vi "发送数组-ccp转换序列.vi"(8 "标定站地址":u32=1 format="%x", 9 "初始地址":u32=15360 format="%x", 10 "输入数组":T2(array[cluster]), 11 "是否剩余":bool) -> (2 "输出数组":T1(array[cluster]) {"Data7" format="%x"; "Data6" format="%x"; "Data5" format="%x"; "Data4" format="%x"; "Data3" format="%x"; "Data2" format="%x"; "Data1" format="%x"; "Data0" format="%x"})   [LabVIEW 2016]
panel:
  in  "CCP命令":u16(ring) items=["CONNECT"=1, "SET_MTA"=2, "DNLOAD"=3, "UPLOAD"=4, "DISCONNECT"=7, "START_STOP_ALL"=8, "SHORT_UPLOAD"=15, "GET_DAQ_SIZE"=20, "SET_DAQ_PTR"=21, "WRITE_DAQ"=22, "EXCHANGE_ID"=23, "DNLOAD6"=35, "UNLOACK"=19, "SET_S_STATUS"=12, "GET_S_STATUS"=13, "SET_CAL_PAGE"=17, "GET_CAL_PAGE"=9, "GET_SEED"=18]
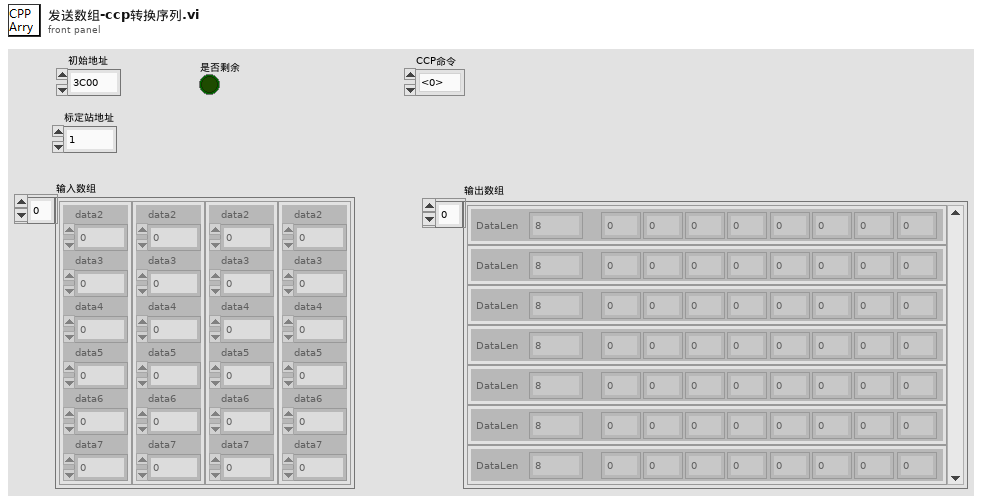
[diagram p1: front panel]
types:
  T1 = cluster{"Data0":u8, "Data1":u8, "Data2":u8, "Data3":u8, "Data4":u8, "Data5":u8, "Data6":u8, "Data7":u8, "DataLen":u8}[]
  T2 = cluster{"data2":u8, "data3":u8, "data4":u8, "data5":u8, "data6":u8, "data7":u8}[]
  T3 = cluster{"Data0":u8, "Data1":u8, "Data2":u8, "Data3":u8, "Data4":u8, "Data5":u8, "Data6":u8, "Data7":u8, "DataLen":u8}
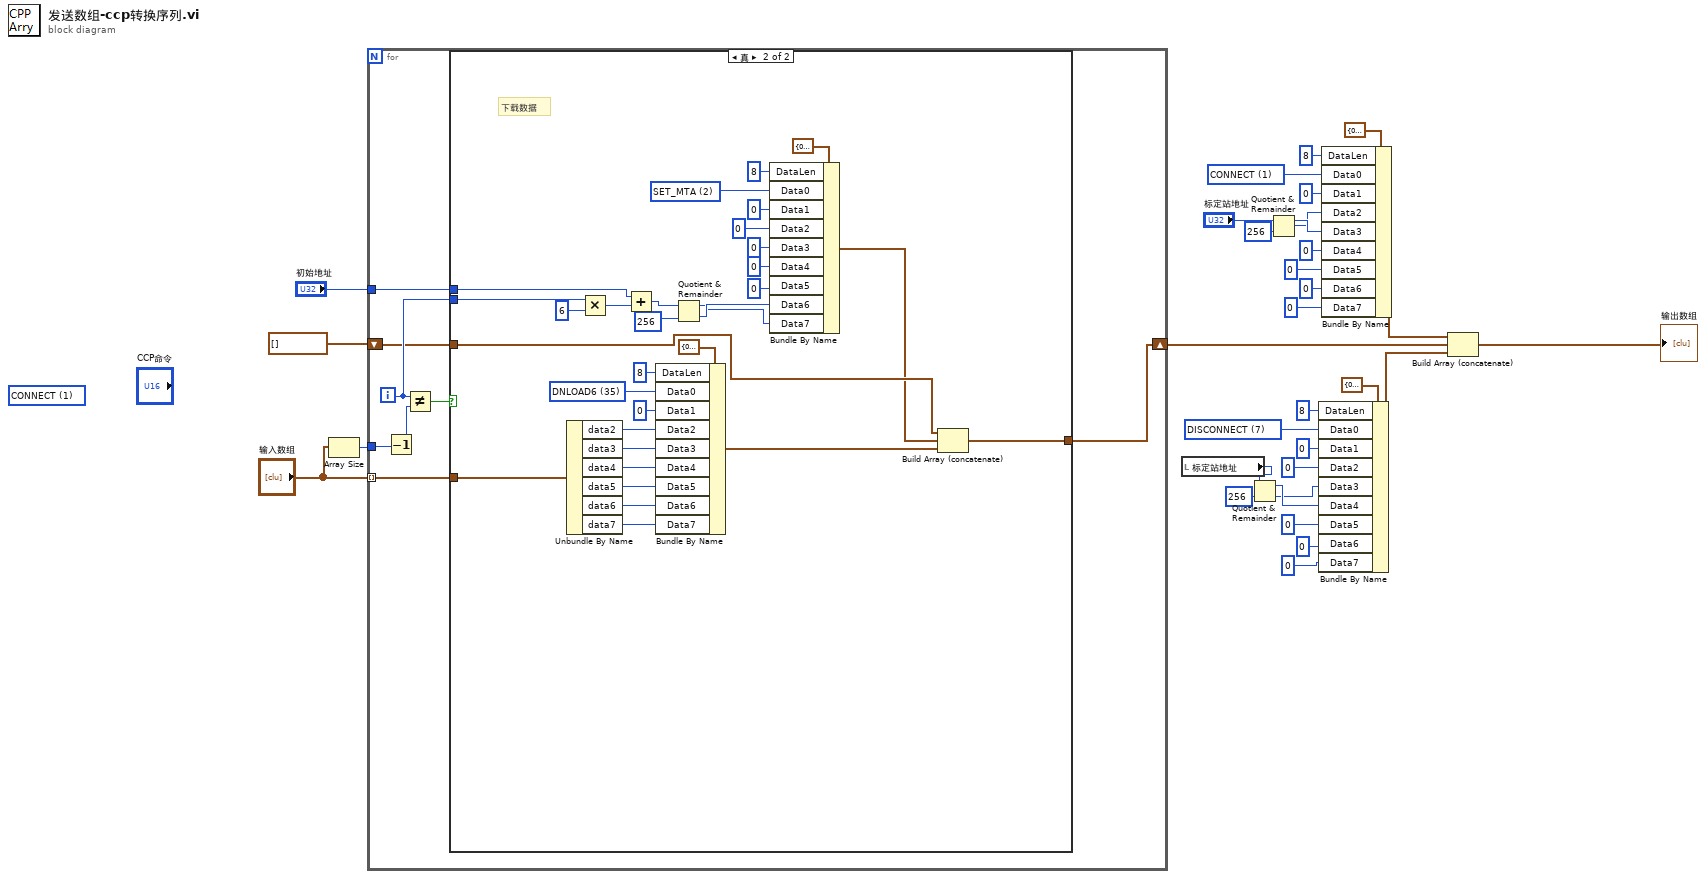
[diagram p0: block diagram]
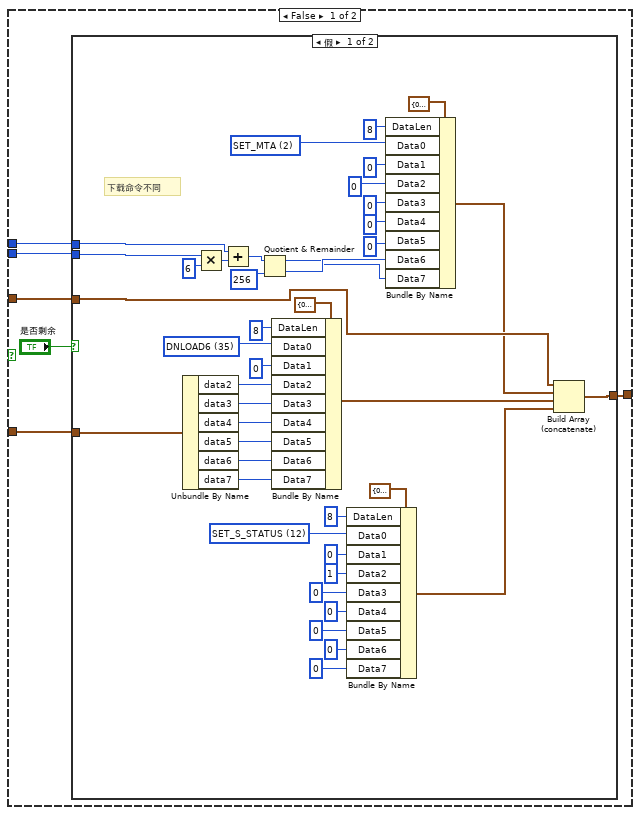
[diagram p2: hidden frame]
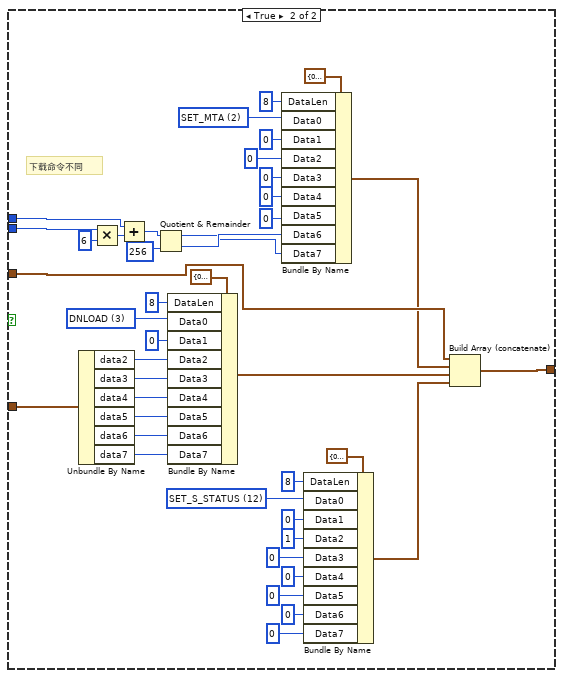
[diagram p3: hidden frame]
diagram:
  w14 = u8 7 items=["CONNECT"=1, "SET_MTA"=2, "DNLOAD"=3, "UPLOAD"=4, "DISCONNECT"=7, "START_STOP_ALL"=8, "SHORT_UPLOAD"=15, "GET_DAQ_SIZE"=20, "SET_DAQ_PTR"=21, "WRITE_DAQ"=22, "EXCHANGE_ID"=23, "DNLOAD6"=35, "UNLOACK"=19, "SET_S_STATUS"=12, "GET_S_STATUS"=13, "SET_CAL_PAGE"=17, "GET_CAL_PAGE"=9, "GET_SEED"=18] ("下拉列表")
  w26 = u8 1 items=["CONNECT"=1, "SET_MTA"=2, "DNLOAD"=3, "UPLOAD"=4, "DISCONNECT"=7, "START_STOP_ALL"=8, "SHORT_UPLOAD"=15, "GET_DAQ_SIZE"=20, "SET_DAQ_PTR"=21, "WRITE_DAQ"=22, "EXCHANGE_ID"=23, "DNLOAD6"=35, "UNLOACK"=19, "SET_S_STATUS"=12, "GET_S_STATUS"=13, "SET_CAL_PAGE"=17, "GET_CAL_PAGE"=9, "GET_SEED"=18] ("下拉列表")
  (unwired) u8 1 items=["CONNECT"=1, "SET_MTA"=2, "DNLOAD"=3, "UPLOAD"=4, "DISCONNECT"=7, "START_STOP_ALL"=8, "SHORT_UPLOAD"=15, "GET_DAQ_SIZE"=20, "SET_DAQ_PTR"=21, "WRITE_DAQ"=22, "EXCHANGE_ID"=23, "DNLOAD6"=35, "UNLOACK"=19, "SET_S_STATUS"=12, "GET_S_STATUS"=13, "SET_CAL_PAGE"=17, "GET_CAL_PAGE"=9, "GET_SEED"=18] ("下拉列表")
  n1 = Array Size(array="输入数组") -> (size(s)=w31:i32)
  n2 = for {
    tunnel: "输入数组" -> [w40] mode=indexing
    tunnel: w31 -> [w34]
    tunnel: "初始地址" -> [w37]
    shift-right: [w35] -> w8
    shift-left: T1 [] -> [w36]
    i -> [w38]
    n3 = Decrement(x=w34) -> (x-1=w33:i32)
    n4 = Not Equal?(x=w38, y=w33) -> (x != y?=w39:bool)
    n5 = case shown="真" w39 {
      tunnel: w40 -> [w45 w161]
      tunnel: w38 -> [w43 w160]
      tunnel: w37 -> [w42 w159]
      tunnel: w36 -> [w44 w158]
      tunnel: [w46 w157] -> w35
      frame False {
        n6 = case shown="假" "是否剩余" {
          tunnel: w45 -> [w87 w130]
          tunnel: w43 -> [w85 w129]
          tunnel: w42 -> [w84 w128]
          tunnel: w44 -> [w86 w127]
          tunnel: [w88 w126] -> w46
          frame False {
            w55 = u8 12 items=["CONNECT"=1, "SET_MTA"=2, "DNLOAD"=3, "UPLOAD"=4, "DISCONNECT"=7, "START_STOP_ALL"=8, "SHORT_UPLOAD"=15, "GET_DAQ_SIZE"=20, "SET_DAQ_PTR"=21, "WRITE_DAQ"=22, "EXCHANGE_ID"=23, "DNLOAD6"=35, "UNLOACK"=19, "SET_S_STATUS"=12, "GET_S_STATUS"=13, "SET_CAL_PAGE"=17, "GET_CAL_PAGE"=9, "GET_SEED"=18] ("下拉列表")
            w59 = u8 35 items=["CONNECT"=1, "SET_MTA"=2, "DNLOAD"=3, "UPLOAD"=4, "DISCONNECT"=7, "START_STOP_ALL"=8, "SHORT_UPLOAD"=15, "GET_DAQ_SIZE"=20, "SET_DAQ_PTR"=21, "WRITE_DAQ"=22, "EXCHANGE_ID"=23, "DNLOAD6"=35, "UNLOACK"=19, "SET_S_STATUS"=12, "GET_S_STATUS"=13, "SET_CAL_PAGE"=17, "GET_CAL_PAGE"=9, "GET_SEED"=18] ("下拉列表")
            w58 = u8 2 items=["CONNECT"=1, "SET_MTA"=2, "DNLOAD"=3, "UPLOAD"=4, "DISCONNECT"=7, "START_STOP_ALL"=8, "SHORT_UPLOAD"=15, "GET_DAQ_SIZE"=20, "SET_DAQ_PTR"=21, "WRITE_DAQ"=22, "EXCHANGE_ID"=23, "DNLOAD6"=35, "UNLOACK"=19, "SET_S_STATUS"=12, "GET_S_STATUS"=13, "SET_CAL_PAGE"=17, "GET_CAL_PAGE"=9, "GET_SEED"=18] ("下拉列表")
            # "下载命令不同"
            n7 = Unbundle By Name(w87) -> ("data2"=w82:u8, "data3"=w81:u8, "data4"=w80:u8, "data5"=w79:u8, "data6"=w78:u8, "data7"=w77:u8)
            n8 = Multiply(x=w85, y=6) -> (x*y=w72:i32)
            n9 = Add(x=w84, y=w72) -> (x+y=w71:u32)
            n10 = Quotient & Remainder(x=w71, y=u32 256) -> (x-y*floor(x/y)=w63:u32, floor(x/y)=w64:u32)
            n11 = Bundle By Name(cluster=T3 {"Data0"=0, "Data1"=0, "Data2"=0, "Data3"=0, "Data4"=0, "Data5"=0, "Data6"=0, "Data7"=0, "DataLen"=8} ("簇 2"), "DataLen"=u8 8, "Data0"=w59, "Data1"=u8 0, "Data2"=w82, "Data3"=w81, "Data4"=w80, "Data5"=w79, "Data6"=w78, "Data7"=w77) -> (w74:T3)
            n12 = Bundle By Name(cluster=T3 {"Data0"=0, "Data1"=0, "Data2"=0, "Data3"=0, "Data4"=0, "Data5"=0, "Data6"=0, "Data7"=0, "DataLen"=8} ("簇 2"), "DataLen"=u8 8, "Data0"=w55, "Data1"=u8 0, "Data2"=u8 1, "Data3"=u8 0, "Data4"=u8 0, "Data5"=u8 0, "Data6"=u8 0, "Data7"=u8 0) -> (w47:T3)
            n13 = Bundle By Name(cluster=T3 {"Data0"=0, "Data1"=0, "Data2"=0, "Data3"=0, "Data4"=0, "Data5"=0, "Data6"=0, "Data7"=0, "DataLen"=8} ("簇 2"), "DataLen"=u8 8, "Data0"=w58, "Data1"=u8 0, "Data2"=u8 0, "Data3"=u8 0, "Data4"=u8 0, "Data5"=u8 0, "Data6"=w64, "Data7"=w63) -> (w60:T3)
            n14 = Build Array (concatenate)(w86, w60, w74, w47) -> (w88:T1)
          }
          frame True {
            w97 = u8 12 items=["CONNECT"=1, "SET_MTA"=2, "DNLOAD"=3, "UPLOAD"=4, "DISCONNECT"=7, "START_STOP_ALL"=8, "SHORT_UPLOAD"=15, "GET_DAQ_SIZE"=20, "SET_DAQ_PTR"=21, "WRITE_DAQ"=22, "EXCHANGE_ID"=23, "DNLOAD6"=35, "UNLOACK"=19, "SET_S_STATUS"=12, "GET_S_STATUS"=13, "SET_CAL_PAGE"=17, "GET_CAL_PAGE"=9, "GET_SEED"=18] ("下拉列表")
            w101 = u8 3 items=["CONNECT"=1, "SET_MTA"=2, "DNLOAD"=3, "UPLOAD"=4, "DISCONNECT"=7, "START_STOP_ALL"=8, "SHORT_UPLOAD"=15, "GET_DAQ_SIZE"=20, "SET_DAQ_PTR"=21, "WRITE_DAQ"=22, "EXCHANGE_ID"=23, "DNLOAD6"=35, "UNLOACK"=19, "SET_S_STATUS"=12, "GET_S_STATUS"=13, "SET_CAL_PAGE"=17, "GET_CAL_PAGE"=9, "GET_SEED"=18] ("下拉列表")
            w100 = u8 2 items=["CONNECT"=1, "SET_MTA"=2, "DNLOAD"=3, "UPLOAD"=4, "DISCONNECT"=7, "START_STOP_ALL"=8, "SHORT_UPLOAD"=15, "GET_DAQ_SIZE"=20, "SET_DAQ_PTR"=21, "WRITE_DAQ"=22, "EXCHANGE_ID"=23, "DNLOAD6"=35, "UNLOACK"=19, "SET_S_STATUS"=12, "GET_S_STATUS"=13, "SET_CAL_PAGE"=17, "GET_CAL_PAGE"=9, "GET_SEED"=18] ("下拉列表")
            # "下载命令不同"
            n15 = Unbundle By Name(w130) -> ("data2"=w124:u8, "data3"=w123:u8, "data4"=w122:u8, "data5"=w121:u8, "data6"=w120:u8, "data7"=w119:u8)
            n16 = Multiply(x=w129, y=6) -> (x*y=w114:i32)
            n17 = Add(x=w128, y=w114) -> (x+y=w113:u32)
            n18 = Quotient & Remainder(x=w113, y=u32 256) -> (x-y*floor(x/y)=w105:u32, floor(x/y)=w106:u32)
            n19 = Bundle By Name(cluster=T3 {"Data0"=0, "Data1"=0, "Data2"=0, "Data3"=0, "Data4"=0, "Data5"=0, "Data6"=0, "Data7"=0, "DataLen"=8} ("簇 2"), "DataLen"=u8 8, "Data0"=w101, "Data1"=u8 0, "Data2"=w124, "Data3"=w123, "Data4"=w122, "Data5"=w121, "Data6"=w120, "Data7"=w119) -> (w116:T3)
            n20 = Bundle By Name(cluster=T3 {"Data0"=0, "Data1"=0, "Data2"=0, "Data3"=0, "Data4"=0, "Data5"=0, "Data6"=0, "Data7"=0, "DataLen"=8} ("簇 2"), "DataLen"=u8 8, "Data0"=w100, "Data1"=u8 0, "Data2"=u8 0, "Data3"=u8 0, "Data4"=u8 0, "Data5"=u8 0, "Data6"=w106, "Data7"=w105) -> (w102:T3)
            n21 = Bundle By Name(cluster=T3 {"Data0"=0, "Data1"=0, "Data2"=0, "Data3"=0, "Data4"=0, "Data5"=0, "Data6"=0, "Data7"=0, "DataLen"=8} ("簇 2"), "DataLen"=u8 8, "Data0"=w97, "Data1"=u8 0, "Data2"=u8 1, "Data3"=u8 0, "Data4"=u8 0, "Data5"=u8 0, "Data6"=u8 0, "Data7"=u8 0) -> (w89:T3)
            n22 = Build Array (concatenate)(w127, w102, w116, w89) -> (w126:T1)
          }
        }
      }
      frame True {
        w132 = u16 2 items=["CONNECT"=1, "SET_MTA"=2, "DNLOAD"=3, "UPLOAD"=4, "DISCONNECT"=7, "START_STOP_ALL"=8, "SHORT_UPLOAD"=15, "GET_DAQ_SIZE"=20, "SET_DAQ_PTR"=21, "WRITE_DAQ"=22, "EXCHANGE_ID"=23, "DNLOAD6"=35, "UNLOACK"=19, "SET_S_STATUS"=12, "GET_S_STATUS"=13, "SET_CAL_PAGE"=17, "GET_CAL_PAGE"=9, "GET_SEED"=18] ("下拉列表")
        w131 = u16 35 items=["CONNECT"=1, "SET_MTA"=2, "DNLOAD"=3, "UPLOAD"=4, "DISCONNECT"=7, "START_STOP_ALL"=8, "SHORT_UPLOAD"=15, "GET_DAQ_SIZE"=20, "SET_DAQ_PTR"=21, "WRITE_DAQ"=22, "EXCHANGE_ID"=23, "DNLOAD6"=35, "UNLOACK"=19, "SET_S_STATUS"=12, "GET_S_STATUS"=13, "SET_CAL_PAGE"=17, "GET_CAL_PAGE"=9, "GET_SEED"=18] ("下拉列表")
        # "下载数据"
        n23 = Unbundle By Name(w161) -> ("data2"=w155:u8, "data3"=w154:u8, "data4"=w153:u8, "data5"=w152:u8, "data6"=w151:u8, "data7"=w150:u8)
        n24 = Multiply(x=w160, y=6) -> (x*y=w145:i32)
        n25 = Add(x=w159, y=w145) -> (x+y=w144:u32)
        n26 = Bundle By Name(cluster=T3 {"Data0"=0, "Data1"=0, "Data2"=0, "Data3"=0, "Data4"=0, "Data5"=0, "Data6"=0, "Data7"=0, "DataLen"=8} ("簇 2"), "DataLen"=u8 8, "Data0"=w131, "Data1"=u8 0, "Data2"=w155, "Data3"=w154, "Data4"=w153, "Data5"=w152, "Data6"=w151, "Data7"=w150) -> (w147:T3)
        n27 = Quotient & Remainder(x=w144, y=u32 256) -> (x-y*floor(x/y)=w136:u32, floor(x/y)=w137:u32)
        n28 = Bundle By Name(cluster=T3 {"Data0"=0, "Data1"=0, "Data2"=0, "Data3"=0, "Data4"=0, "Data5"=0, "Data6"=0, "Data7"=0, "DataLen"=8} ("簇 2"), "DataLen"=u8 8, "Data0"=w132, "Data1"=u8 0, "Data2"=u8 0, "Data3"=u8 0, "Data4"=u8 0, "Data5"=u8 0, "Data6"=w137, "Data7"=w136) -> (w133:T3)
        n29 = Build Array (concatenate)(w158, w133, w147) -> (w157:T1)
      }
    }
  }
  n30 = local read "标定站地址"() -> (w1:u32)
  n31 = Quotient & Remainder(x=w1, y=u32 256) -> (x-y*floor(x/y)=w3:u32, floor(x/y)=w2:u32)
  n32 = Quotient & Remainder(x="标定站地址", y=u32 256) -> (x-y*floor(x/y)=w18:u32, floor(x/y)=w17:u32)
  n33 = Bundle By Name(cluster=T3 {"Data0"=0, "Data1"=0, "Data2"=0, "Data3"=0, "Data4"=0, "Data5"=0, "Data6"=0, "Data7"=0, "DataLen"=8} ("簇 2"), "DataLen"=u8 8, "Data0"=w14, "Data1"=u8 0, "Data2"=u8 0, "Data3"=w2, "Data4"=w3, "Data5"=u8 0, "Data6"=u8 0, "Data7"=u8 0) -> (w6:T3)
  n34 = Bundle By Name(cluster=T3 {"Data0"=0, "Data1"=0, "Data2"=0, "Data3"=0, "Data4"=0, "Data5"=0, "Data6"=0, "Data7"=0, "DataLen"=8} ("簇 2"), "DataLen"=u8 8, "Data0"=w26, "Data1"=u8 0, "Data2"=w17, "Data3"=w18, "Data4"=u8 0, "Data5"=u8 0, "Data6"=u8 0, "Data7"=u8 0) -> (w7:T3)
  n35 = Build Array (concatenate)(w7, w8, w6) -> (→"输出数组":T1)
